vi "LHF.DB.Mongo.Bson.Timestamp.vi"(0 "t0":timestamp, 5 "error in (no error)":errorcluster) -> (14 "BsonString":refnum<k24>, 19 "error out":errorcluster)   [LabVIEW 2013, in "LHF.DB.Mongo.lvclass"]
uses:
  LHF.DB.Mongo.lvclass
  C:/Users/Ricardo/Desktop/Projetos/LabVIEW-MongoDB/src/Driver/MongoDB.Bson.dll
  LabVIEW-MongoDB/src/Driver/MongoDB.Bson.dll
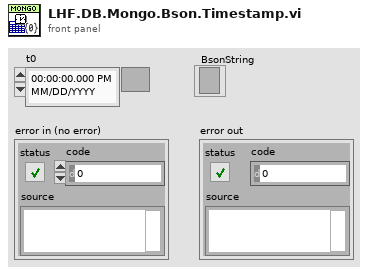
[diagram p1: front panel]
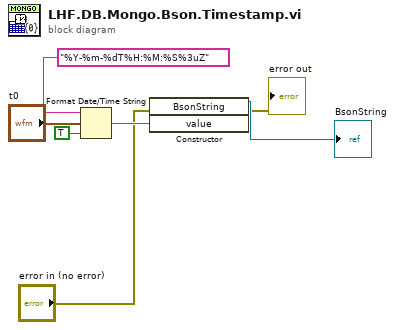
[diagram p0: block diagram]
diagram:
  n1 = Format Date/Time String(time format string (%c)="%Y-%m-%dT%H:%M:%S%3uZ", seconds (now)="t0", UTC format=TRUE) -> (date/time string=w3:string)
  n2 = constructor class="BsonString"(error in="error in (no error)", "value"=w3) -> (reference out=→"BsonString":refnum<k24>, error out=→"error out":errorcluster)  [unwired: 2 in, 2 out]
